vi "transfer_hadamard_to_DLP_NR_mk3_.vi"(6 "Progress Indicator":refnum<vi>, 8 "error in (no error)":errorcluster, 9 "Hadamard":bool[][](array[boolean]), 10 "SequenceId":u32, 11 "DeviceId":u32) -> (0 "error out":errorcluster, 2 "SequenceId Out":u32, 3 "DeviceId Out":u32)   [LabVIEW 2020]
uses:
  upscale_array.vi
  <vilib>/Analysis/baseanly.llb/Mean.vi
  <vilib>/Analysis/baseanly.llb/Mean (DBL).vi
  <vilib>/Utility/error.llb/Error Cluster From Error Code.vi
  <userlib>/alp4395/alp4395.dll
panel:
  out "size(s)":i32[](array[numeric])
  out "Total Frames":i32
  out "Progress":dbl(slide) scale=0.0..1.0
  out "Frames Transferred":i32
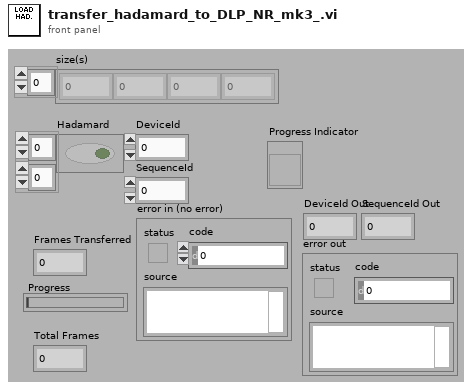
[diagram p1: front panel]
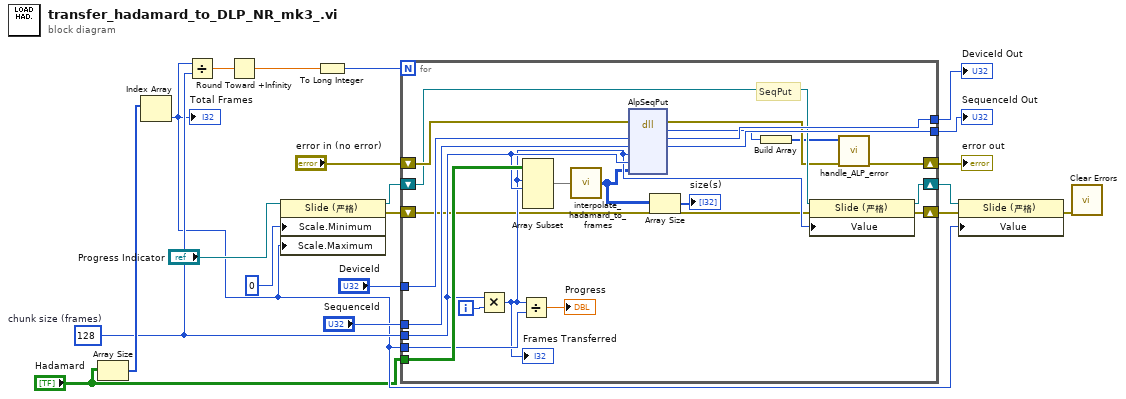
[diagram p0: block diagram]
diagram:
  w10 = 128  # chunk size (frames)
  n1 = Array Size(array="Hadamard") -> (size(s)=w18:i32[])
  n2 = Index Array(array=w18) -> (element=w4:i32)  [unwired: 1 in]
  "Total Frames" <- w4
  n3 = Divide(x=w4, y=w10) -> (x/y=w17:dbl)
  n4 = Round Toward +Infinity(x=w17) -> (ceil(x): smallest int >= x=w16:dbl)
  n5 = property class="Slide (严格)"(reference="Progress Indicator", "Scale.Minimum"=0 ("element"), "Scale.Maximum"=w4) -> (reference out=w7:refnum<vi>, error out=w5:errorcluster)  [unwired: 1 in]
  n6 = To Long Integer(number=w16) -> (32bit integer=w15:i32)
  n7 = for {
    N: w15 -> [_]
    tunnel: "DeviceId" -> [w42]
    tunnel: "SequenceId" -> [w41]
    tunnel: "Hadamard" -> [w40]
    tunnel: w10 -> [w39]
    tunnel: w4 -> [w34]
    tunnel: [w37] -> w14
    tunnel: [w36] -> w13
    shift-right: [w27] -> w11
    shift-left: "error in (no error)" -> [w35]
    shift-right: [w30] -> w6
    shift-left: w7 -> [w32]
    shift-right: [w28] -> w3
    shift-left: w5 -> [w29]
    i -> [w33]
    # "SeqPut"
    n8 = Multiply(x=w39, y=w33) -> (x*y=w31:i32)
    "Frames Transferred" <- w31
    n9 = Divide(x=w31, y=w34) -> (x/y=→"Progress":dbl)
    n10 = Array Subset(array=w40, index (row)=w31, length (row)=w39) -> (w23:bool[][])  [unwired: 2 in]
    n11 = call "interpolate_hadamard_to_frames.vi"("Hadamard"=w23) -> ("Fames"=w22:u8[][][])
    n12 = dll-call lib="C:/Program Files (x86)/National Instruments/LabVIEW 2020/user.lib/alp4395/alp4395.dll" fn="AlpSeqPut"(error in=w35, "DeviceId"=w42, "SequenceId"=w41, "PicOffset"=w31, "PicLoad"=w39, "UserArrayPtr"=w22) -> (error out=w26:errorcluster, "return type"=w24:i32, "DeviceId"=w37:u32, "SequenceId"=w36:u32)  [unwired: 5 in, 1 out]
    n13 = Array Size(array=w22) -> (size(s)=→"size(s)":i32[])
    n14 = Build Array(w24) -> (w25:i32[])
    n15 = property class="Slide (严格)"(reference=w32, error in=w29, "Value"=w31) -> (reference out=w30:refnum<vi>, error out=w28:errorcluster)
    n16 = call "handle_ALP_error.vi"("error in"=w26, "Return Codes"=w25) -> ("error out"=w27:errorcluster)  [unwired: 9 in]
  }
  "DeviceId Out" <- w14
  "SequenceId Out" <- w13
  "error out" <- w11
  n17 = property class="Slide (严格)"(reference=w6, error in=w3, "Value"=w4) -> (error out=w2:errorcluster)  [unwired: 1 out]
  n18 = call <vilib>:"Clear Errors.vi"("error in (no error)"=w2) -> ()  [unwired: 5 in, 2 out]
